vi "driveTurn.vi"(10 "fwd direction":dbl, 11 "hdg target":dbl) -> ()   [LabVIEW 2011]
uses:
  common/scale_const.ctl
  drivetrain/gear_shift_state.ctl
  drivetrain/drivetrain_drive_mode.ctl
  drivetrain/drivetrain_drive_write_thread.ctl
  Auto_Conf.vi
  drivetrain/drivetrain_globals.vi
panel:
  in  "integral cap":T1={"min_ana"=0.0, "min_units"=5.0, "max_ana"=45.0, "max_units"=0.0}
  out "error":dbl(graph)
  out "angle":dbl
  in  "hdg kI":dbl=0.005
  in  "hdg kP":dbl=0.09
  out "x > y?":bool
  in  "max speed":dbl=12.0
  in  "speed_kI":dbl=-0.005
  in  "speed_kP":dbl=-0.4
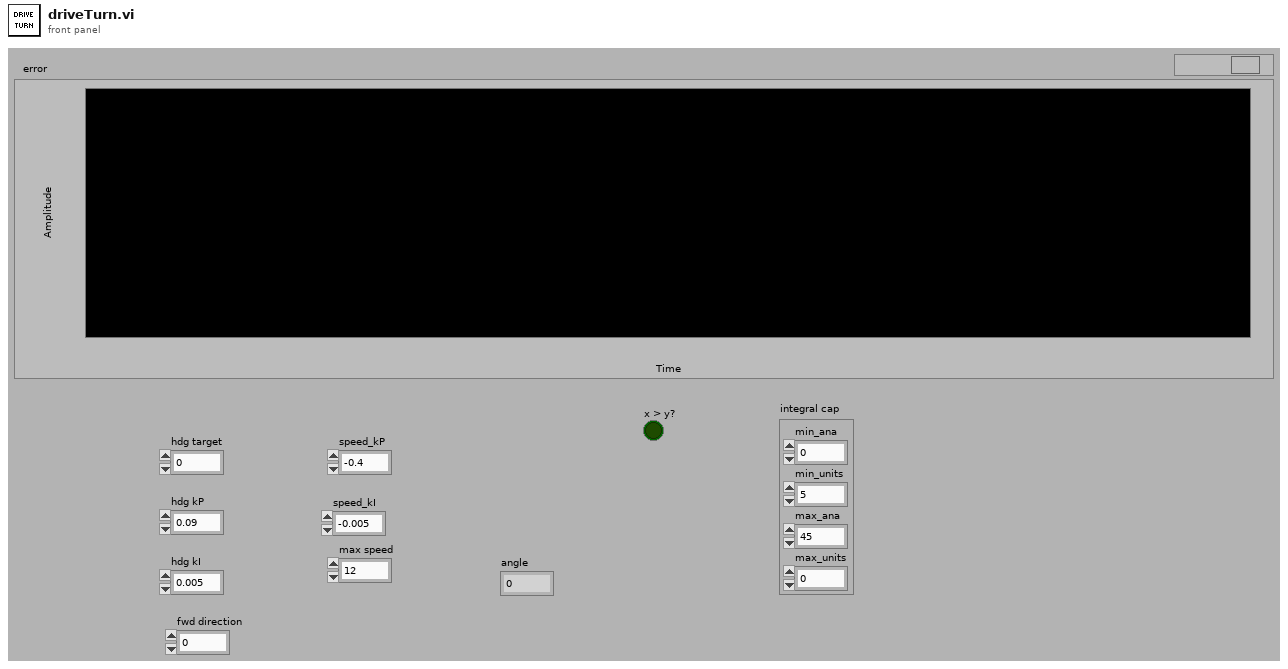
[diagram p1: front panel]
types:
  T1 = typedef "scale_const.ctl" = cluster{"min_ana":dbl, "min_units":dbl, "max_ana":dbl, "max_units":dbl}
  T2 = typedef "WPI_GyroDevRef.ctl" = cluster{"DevStatus":errorcluster, "Analog Module":T3, "Analog Channel":T4, "Offset":dbl, "Gain (VoltsPerDegree/Second)":dbl}
  T3 = typedef "FPGA_TypedefAnalogModule.ctl" = enum16{"Analog Module 1", "Analog Module 2"}
  T4 = typedef "FPGA_AIChannel.ctl" = enum8{"AI 1", "AI 2", "AI 3", "AI 4", "AI 5", "AI 6", "AI 7", "AI 8", "Invalid"}
  T5 = typedef "gear_shift_state.ctl" = enum16{"low", "high"}
  T6 = typedef "drivetrain_drive_mode.ctl" = enum16{"open loop", "closed loop"}
  T7 = typedef "drivetrain_drive_write_thread.ctl" = enum16{"Teleop", "Script Engine - Autonomous", "Script Engine - Sequence"}
  T8 = typedef "WPI_RobotDriveDevRef.ctl" = cluster{"DevStatus":errorcluster, "Motors[]":T9[], "Square Inputs":bool, "Max Output":dbl}
  T9 = typedef "WPI_MotorControlDeviceRef.ctl" = cluster{"DeviceStatus":errorcluster, "Type":enum16{"PWM", "CAN"}, "PWM":cluster{"Digital Module":T10, "PWM Channel":T11, "DeadBand":T12}, "CAN":cluster{"Device Number":u8, "Control Mode":T13, "Semaphore":T14, "Max Vout":dbl}, "Invert":bool, "TransformRef":T15, "InvTransformRef":T15}
  T10 = typedef "FPGA_TypedefDigitalModule.ctl" = enum16{"Digital Module 1", "Digital Module 2"}
  T11 = typedef "FPGA_DIOPWMChannel.ctl" = enum8{"PWM 1", "PWM 2", "PWM 3", "PWM 4", "PWM 5", "PWM 6", "PWM 7", "PWM 8", "PWM 9", "PWM 10", "Invalid"}
  T12 = typedef "WPI_PWMDeadband.ctl" = cluster{"Name":string, "maxPositivePwm":i32, "minPositivePwm":i32, "centerPwm":i32, "maxNegativePwm":i32, "minNegativePwm":i32, "angularRange":u16}
  T13 = typedef "WPI_CANJaguar_ControlMode.ctl" = enum8{"Percent VBus", "Current", "Speed", "Position", "Voltage"}
  T14 = typedef "Semaphore RefNum" = refnum<k1>
  T15 = typedef "WPI_PWMTransform_ConPane.ctl" = refnum<vi>
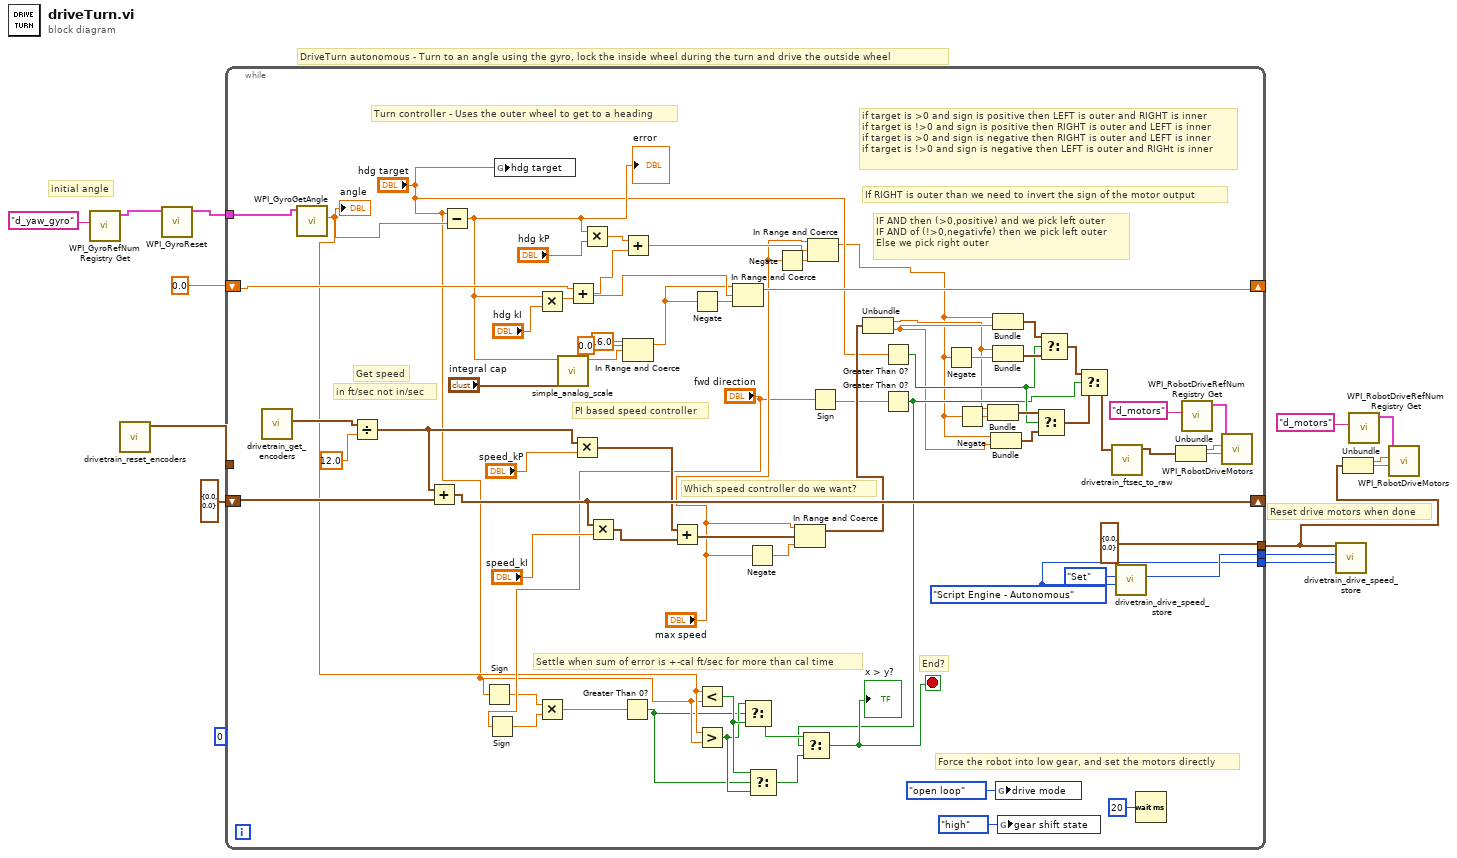
[diagram p0: block diagram]
diagram:
  (unwired) u32 0
  # "initial angle"
  # "DriveTurn autonomous - Turn to an angle using the gyro, lock the inside wheel during the turn and drive the outside wheel"
  # "Reset drive motors when done"
  n1 = call <vilib>:"WPI_GyroRefNum Registry Get.vi"("refnum name"="d_yaw_gyro") -> ("GyroDevRef"=w2:T2)  [unwired: 1 in, 9 out]
  n2 = call "drivetrain_reset_encoders.vi"() -> ("Distance (in)"=w13:cluster{"Left":dbl, "Right":dbl})  [unwired: 9 in, 2 out]
  n3 = call <vilib>:"WPI_GyroReset.vi"("GyroDevRef"=w2) -> ("GyroDevRef"=w1:T2)  [unwired: 9 in, 1 out]
  n4 = while {
    tunnel: w13 -> [_]
    tunnel: [cluster{"Left":dbl, "Right":dbl} {"Left"=0.0, "Right"=0.0} ("Drive")] -> w8
    tunnel: [w79] -> w12
    tunnel: [w78] -> w11
    shift-right: [w66] -> _
    shift-left: cluster{"Left":dbl, "Right":dbl} {"Left"=0.0, "Right"=0.0} -> [w67]
    shift-right: [w55] -> _
    shift-left: 0.0 -> [w47]
    tunnel: w1 -> [w58]
    stop <- w20 stop-if-true
    w78 = drivetrain_drive_write_thread."Script Engine - Autonomous" ("Write Thread")
    w79 = enum16{"Set", "Get"}."Set" ("data_store_mode")
    # "IF AND then (>0,positive) and we pick left outer\nIF AND of (!>0,negativfe) then we pick left outer\nElse we pick right outer"
    # "If RIGHT is outer than we need to invert the sign of the motor output"
    # "if target is >0 and sign is positive then LEFT is outer and RIGHT is inner\nif target is !>0 and sign is positive then RIGHT is outer and LEFT is inner\nif target is >0 and sign is negative then RIGHT is outer and LEFT is inner\nif target is !>0 and sign is negative then LEFT is outer and RIGHt is inner"
    # "Which speed controller do we want?"
    # "Turn controller - Uses the outer wheel to get to a heading"
    # "Settle when sum of error is +-cal ft/sec for more than cal time"
    # "PI based speed controller"
    # "in ft/sec not in/sec"
    # "Get speed"
    # "End?"
    # "Force the robot into low gear, and set the motors directly"
    n5 = call "drivetrain_get_encoders.vi"() -> ("Velocity (in/sec)"=w70:cluster{"Left":dbl, "Right":dbl})  [unwired: 9 in, 2 out]
    n6 = call <vilib>:"WPI_GyroGetAngle.vi"("GyroDevRef"=w58) -> ("Angle"=w33:dbl)  [unwired: 1 in, 9 out]
    "angle" <- w33
    n7 = Divide(x=w70, y=12.0) -> (x/y=w60:cluster{"Left":dbl, "Right":dbl})
    n8 = Add(x=w60, y=w67) -> (x+y=w66:cluster{"Left":dbl, "Right":dbl})
    n9 = Subtract(x="hdg target", y=w33) -> (x-y=w44:dbl)
    "error" <- w44
    n10 = Sign(1:"hdg target") -> (0:w36:dbl)
    n11 = Sign(1:"fwd direction") -> (0:w35:dbl)
    n12 = global write "Auto_Conf.vi" "hdg target"("hdg target") -> ()
    n13 = Multiply(x=w44, y="hdg kI") -> (x*y=w46:dbl)
    n14 = Multiply(x=w36, y=w35) -> (x*y=w34:dbl)
    n15 = call "simple_analog_scale.vi"("Scale Const"="integral cap", "Analog"=w44) -> ("Units"=w42:dbl)  [unwired: 9 in]
    n16 = Add(x=w47, y=w46) -> (x+y=w45:dbl)
    n17 = Multiply(x=w60, y="speed_kP") -> (x*y=w64:cluster{"Left":dbl, "Right":dbl})
    n18 = Multiply(x=w44, y="hdg kP") -> (x*y=w53:dbl)
    n19 = Multiply(x=w66, y="speed_kI") -> (x*y=w63:cluster{"Left":dbl, "Right":dbl})
    n20 = Greater Than 0?(x=w34) -> (x > 0?=w23:bool)
    n21 = Add(x=w53, y=w45) -> (x+y=w50:dbl)
    n22 = In Range and Coerce(upper limit=16.0, x=w42, lower limit=0.0) -> (coerced(x)=w39:dbl)  [unwired: 1 out]
    n23 = Add(x=w64, y=w63) -> (x+y=w62:cluster{"Left":dbl, "Right":dbl})
    n24 = Negate(x=w39) -> (-x=w56:dbl)
    n25 = Less?(x=w33, y="hdg target") -> (x < y?=w25:bool)
    n26 = Greater?(x=w33, y="hdg target") -> (0:w24:bool)
    n27 = In Range and Coerce(upper limit=w39, x=w45, lower limit=w56) -> (coerced(x)=w55:dbl)  [unwired: 1 out]
    n28 = Select(t=w24, s=w23, f=w25) -> (s? t:f=w22:bool)
    n29 = Negate(x="max speed") -> (-x=w61:dbl)
    n30 = Select(t=w25, s=w23, f=w24) -> (s? t:f=w21:bool)
    n31 = Negate(x="max speed") -> (-x=w49:dbl)
    n32 = In Range and Coerce(upper limit="max speed", x=w62, lower limit=w61) -> (coerced(x)=w59:cluster{"Left":dbl, "Right":dbl})  [unwired: 1 out]
    n33 = In Range and Coerce(upper limit="max speed", x=w50, lower limit=w49) -> (coerced(x)=w14:dbl)  [unwired: 1 out]
    n34 = Sign(1:"fwd direction") -> (0:w31:dbl)
    n35 = Unbundle(w59) -> ("Left"=w16:dbl, "Right"=w17:dbl)
    n36 = Greater Than 0?(x="hdg target") -> (x > 0?=w26:bool)
    n37 = Greater Than 0?(x=w31) -> (x > 0?=w19:bool)
    n38 = Select(t=w22, s=w19, f=w21) -> (s? t:f=w20:bool)
    "x > y?" <- w20
    n39 = Negate(x=w14) -> (-x=w38:dbl)
    n40 = Negate(x=w14) -> (-x=w15:dbl)
    n41 = Bundle("Left"=w16, w15) -> (w28:cluster{"Left":dbl, dbl})  [unwired: 1 in]
    n42 = Bundle("max speed"=w14, "Right"=w17) -> (w27:cluster{"max speed":dbl, "Right":dbl})  [unwired: 1 in]
    n43 = Bundle("max speed"=w14, "Right"=w17) -> (w52:cluster{"max speed":dbl, "Right":dbl})  [unwired: 1 in]
    n44 = Bundle("Left"=w16, w38) -> (w51:cluster{"Left":dbl, dbl})  [unwired: 1 in]
    n45 = global write "drivetrain_globals.vi" "drive mode"(drivetrain_drive_mode."open loop" ("drive mode")) -> ()
    n46 = global write "drivetrain_globals.vi" "gear shift state"(gear_shift_state."high" ("gear shift state")) -> ()
    n47 = Select(t=w28, s=w26, f=w27) -> (s? t:f=w18:cluster{"max speed":dbl, "Right":dbl})
    n48 = Select(t=w52, s=w26, f=w51) -> (s? t:f=w29:cluster{"Left":dbl, "Right":dbl})
    n49 = Select(t=w29, s=w19, f=w18) -> (s? t:f=w30:cluster{"max speed":dbl, "Right":dbl})
    n50 = call "drivetrain_ftsec_to_raw.vi"("Drive Data"=w30) -> ("Drive Data Out"=w71:cluster{"Left":dbl, "Right":dbl})  [unwired: 10 in]
    n51 = call "drivetrain_drive_speed_store.vi"("Write Thread"=w78, "data_store_mode"=w79) -> ()  [unwired: 8 in, 2 out]
    n52 = Wait (ms)(milliseconds to wait=u32 20) -> ()  [unwired: 1 out]
    n53 = Unbundle(w71) -> ("Left"=w73:dbl, "Right"=w74:dbl)
    n54 = call <vilib>:"WPI_RobotDriveRefNum Registry Get.vi"("refnum name"="d_motors") -> ("RobotDriveDevRef"=w76:T8)  [unwired: 9 in, 1 out]
    n55 = call <vilib>:"WPI_RobotDriveMotors.vi"("RightSpeed"=w74, "LeftSpeed"=w73, "RobotDriveDevRef"=w76) -> ()  [unwired: 7 in, 2 out]
  }
  n56 = call "drivetrain_drive_speed_store.vi"("Write Thread"=w11, "data_store_mode"=w12, "drive data"=w8) -> ()  [unwired: 7 in, 2 out]
  n57 = Unbundle(w8) -> ("Left"=w10:dbl, "Right"=w9:dbl)
  n58 = call <vilib>:"WPI_RobotDriveRefNum Registry Get.vi"("refnum name"="d_motors") -> ("RobotDriveDevRef"=w6:T8)  [unwired: 9 in, 1 out]
  n59 = call <vilib>:"WPI_RobotDriveMotors.vi"("RightSpeed"=w9, "LeftSpeed"=w10, "RobotDriveDevRef"=w6) -> ()  [unwired: 7 in, 2 out]
